vi "Card Read.vi"(8 "error in":errorcluster, 10 "Data":variant) -> (0 "error out":errorcluster)   [LabVIEW 2013, in "Display Console.lvlib"]
doc: "This VI enqueues the named action."
uses:
  Display Console.lvlib
  Private Controls/Module Data Cluster.ctl
  Private Controls/Display Action.ctl
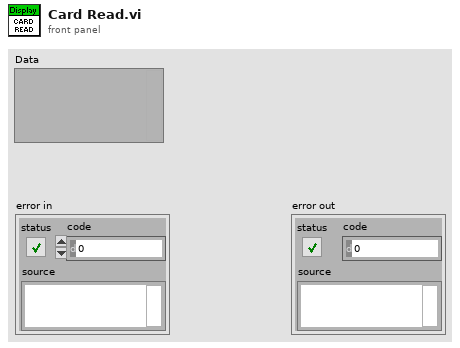
[diagram p1: front panel]
types:
  T1 = typedef "Display Console.lvlib/Module Data Cluster.ctl" = cluster{"Data":variant, "Action":T2}
  T2 = typedef "Display Console.lvlib/Display Action.ctl" = enum16{"Init", "Message", "Transaction", "Card", "Exit", "Error"}
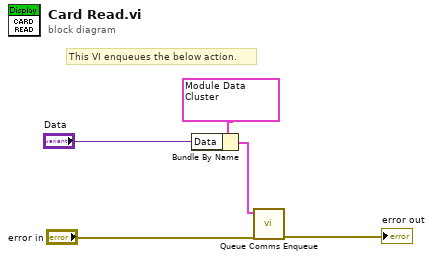
[diagram p0: block diagram]
diagram:
  # "This VI enqueues the below action."
  n1 = Bundle By Name(cluster=T1 {"Data"=variant, "Action"=enum."Card"} ("element"), "Data"="Data") -> (w2:T1)
  n2 = call "Queue Comms Enqueue.vi"("error in"="error in", "element"=w2) -> ("error out"=→"error out":errorcluster)  [unwired: 9 in]
